vi "VdAnalogInput_DAQmx_Create.vi"(6 "VoltageRangeHigh":dbl, 8 "Error In":errorcluster, 9 "VoltageRangeLow":dbl, 10 "Address":string, 11 "reference in":refnum<class "VdAnalogInput_DAQmx.lvclass">) -> (0 "Error Out":errorcluster, 3 "reference out":refnum<class "VdAnalogInput_DAQmx.lvclass">)   [LabVIEW 2020, in "VdAnalogInput_DAQmx.lvclass"]
uses:
  VdAnalogInput_DAQmx.lvclass
  VdAnalogInput_DAQmx.lvclass/VdAnalogInput_DAQmx.ctl
  VdAnalogInput_class/VdAnalogInput.lvclass
  <vilib>/DAQmx/create/channels.llb/DAQmx Create Channel (AI-Voltage-Basic).vi
  C:/Projects/OpenGDS_DesignPatterns/Factory1/VdAnalogInput_class/VdAnalogInput.lvclass
  C:/Projects/OpenGDS_DesignPatterns/Factory1/VdInstrument_class/VdInstrument.lvclass
  C:/Projects/OpenGDS_DesignPatterns/Factory1/VdAnalogInput_DAQmx_class/VdAnalogInput_DAQmx.lvclass
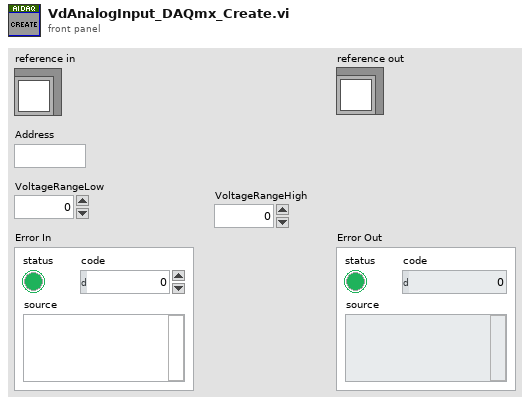
[diagram p1: front panel]
types:
  T1 = typedef "VdAnalogInput_DAQmx.lvclass/ObjectAttributes.ctl" = cluster{"task":refnum<k21>}
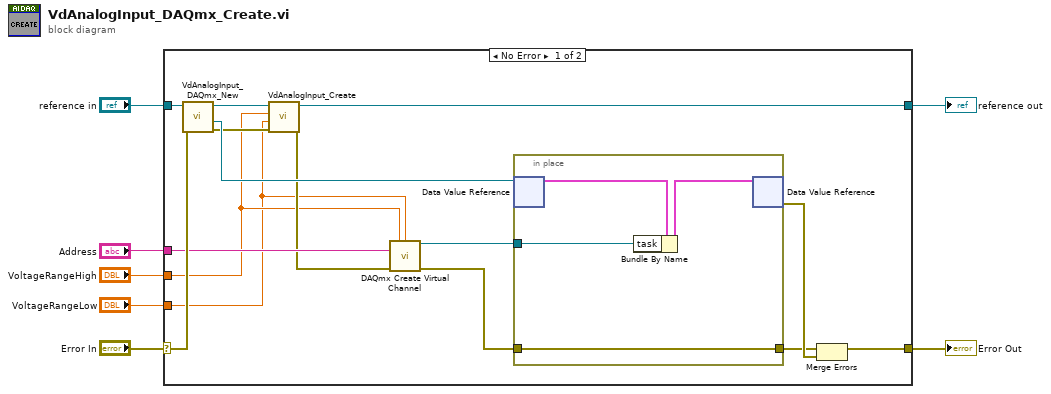
[diagram p0: block diagram]
diagram:
  n1 = case shown="No Error" "Error In" {
    selector: "Error In" -> [w18 w28]
    tunnel: [w16 w28] -> w6
    tunnel: "reference in" -> [w20 w27]
    tunnel: [w15 w27] -> w4
    tunnel: "Address" -> [w13 _]
    tunnel: "VoltageRangeLow" -> [w8 _]
    tunnel: "VoltageRangeHigh" -> [w9 _]
    frame No Error {
      n2 = call "VdAnalogInput_DAQmx_New.vi"("error in (no error)"=w18, "reference in"=w20) -> ("error out"=w19:errorcluster, "DVRRefOut"=w22:refnum<data-value>, "reference out"=w21:refnum<class "VdAnalogInput_DAQmx.lvclass">)  [unwired: 6 in, 1 out]
      n3 = call "VdAnalogInput_Create.vi"("Error In"=w19, "VoltageRangeLow"=w8, "VoltageRangeHigh"=w9, "reference in"=w21) -> ("Error Out"=w12:errorcluster, "reference out"=w15:refnum<class "VdAnalogInput_DAQmx.lvclass">)  [unwired: 6 in]
      n4 = call-poly <vilib>:"DAQmx Create Virtual Channel.vi"("maximum value"=w9, "minimum value"=w8, "physical channels"=w13, "error in"=w12) -> ("task out"=w10:refnum<k21>, "error out"=w11:errorcluster)  [unwired: 10 in]
      n5 = in-place {
        in-place-border: w11 -> [w26]
        in-place-border: [w26] -> w14
        in-place-border: w10 -> [w23]
        n6 = in-place-dvr #1(w22) -> (w25:T1)  [unwired: 1 out]
        n7 = Bundle By Name(cluster=w25, "task"=w23) -> (w24:T1)
        n8 = in-place-dvr #1(w24) -> (w17:errorcluster)  [unwired: 1 out]
      }
      n9 = Merge Errors(w14, w17) -> (w16:errorcluster)
    }
    frame Error {
    }
  }
  "Error Out" <- w6
  "reference out" <- w4
